vi "test Get Blob Service Stats.vi"(8 "error in (no error)":errorcluster, 11 "TestCase in":refnum<class "Test_Blob.lvclass">) -> (0 "error out":errorcluster, 3 "TestCase out":refnum<class "Test_Blob.lvclass">)   [LabVIEW 2015, in "Test_Blob.lvclass"]
uses:
  Test_Blob.lvclass
  Global Parameters.vi
  Core/Session/Session.lvclass
  Blob Storage/NI_Azure_Blob.lvlib
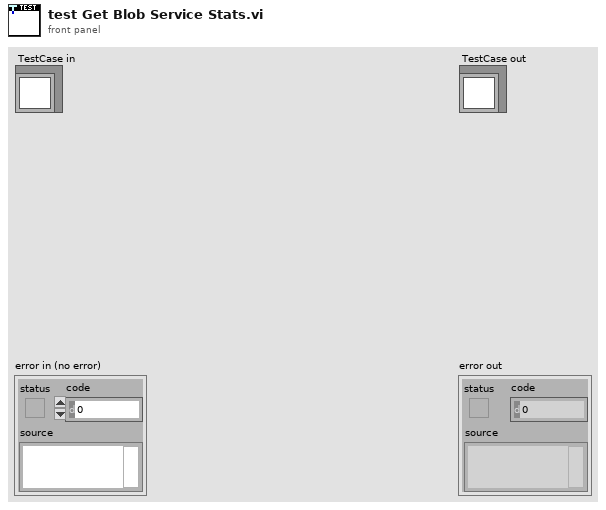
[diagram p1: front panel]
types:
  T1 = typedef "NI_Azure_Core.lvlib/Session.lvclass/Azure Credentials.ctl" = cluster{"Storage Account Name":string, "Access Key":string}
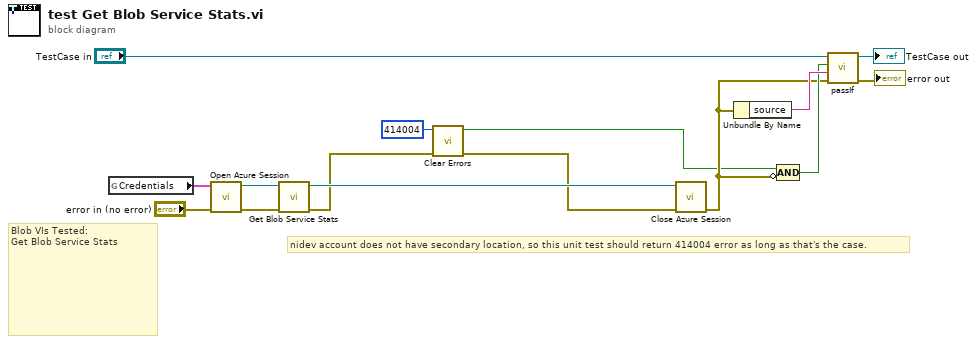
[diagram p0: block diagram]
diagram:
  # "nidev account does not have secondary location, so this unit test should return 414004 error as long as that's the case."
  # "Blob VIs Tested:\nGet Blob Service Stats"
  n1 = global read "Global Parameters.vi" "Credentials"() -> (w10:T1)
  n2 = call "Open Azure Session.vi"("error in (no error)"="error in (no error)", "Credentials"=w10) -> ("error out"=w7:errorcluster, "Azure Session"=w8:refnum<class "Session.lvclass">)  [unwired: 8 in]
  n3 = call "Get Blob Service Stats.vi"("error in (no error)"=w7, "Azure Session in"=w8) -> ("error out"=w5:errorcluster, "Azure Session out"=w6:refnum<class "Session.lvclass">)  [unwired: 6 in, 2 out]
  n4 = call <vilib>:"Clear Errors.vi"("error in (no error)"=w5, "specific error code to clear (0: all)"=414004) -> ("error out"=w3:errorcluster, "specific error cleared?"=w2:bool)  [unwired: 4 in]
  n5 = call "Close Azure Session.vi"("error in (no error)"=w3, "Azure Session"=w6) -> ("error out"=w4:errorcluster)  [unwired: 9 in]
  n6 = Unbundle By Name(w4) -> ("source"=w12:string)
  n7 = Compound Arithmetic op=AND(w2, invert w4) -> (w9:bool)
  n8 = call-dynamic "passIf.vi"("error in (no error)"=w4, "message (\"\")"=w12, "pass"=w9, "TestCase in"="TestCase in") -> ("error out"=→"error out":errorcluster, "TestCase out"=→"TestCase out":refnum<class "Test_Blob.lvclass">)  [unwired: 6 in]
